vi "Get Package Available Versions.vi"(8 "error in":errorcluster, 11 "package name":string) -> (0 "error out":errorcluster, 2 "versions":string[](array[string]), 3 "package name out":string)   [LabVIEW 2014, in "NIPM_API.lvlib"]
doc: "Returns a list of all the versions (from highest to lowest) of the specified package (in all currently registered feeds on this computer)\n\nINPUT(s)\n<B>Package name</B>: Specifies the package\n\nOUTPUT(s)\n<B>Package name out</B>: Outputs the package name\n\n<B>Versions</B>: Outputs a 1D array that lists all of the available versions of the package from highest to lowest"
uses:
  NIPM_API.lvlib
panel:
  out "cmd standard output":string
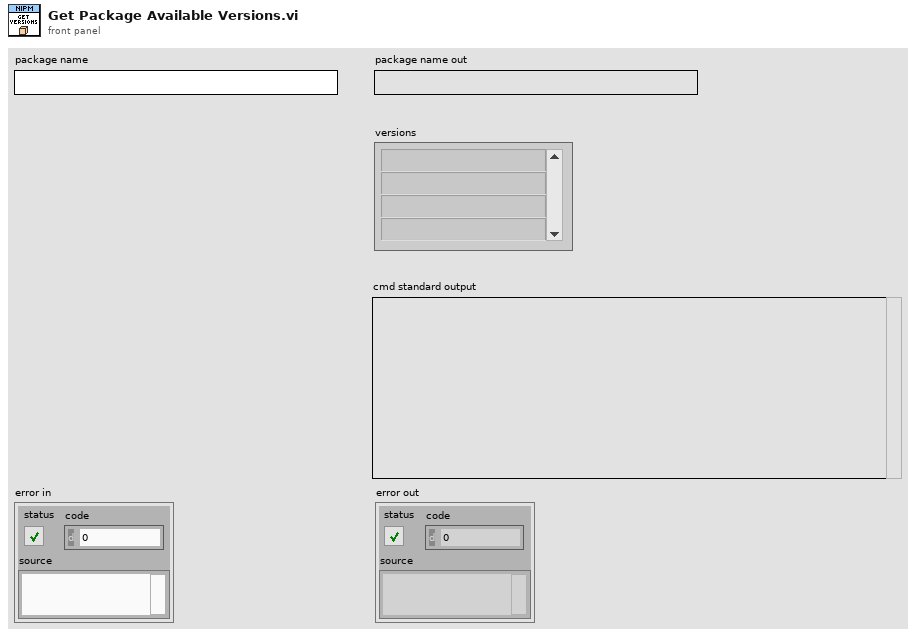
[diagram p1: front panel]
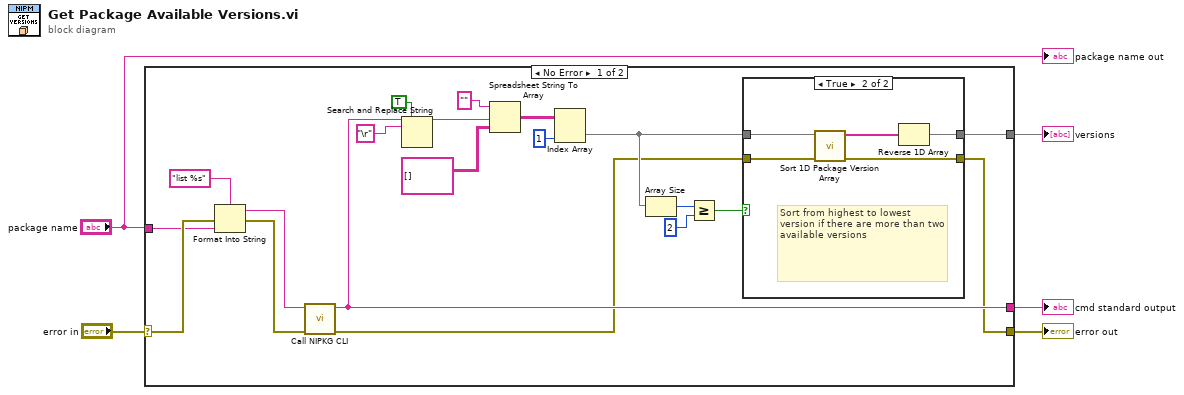
[diagram p0: block diagram]
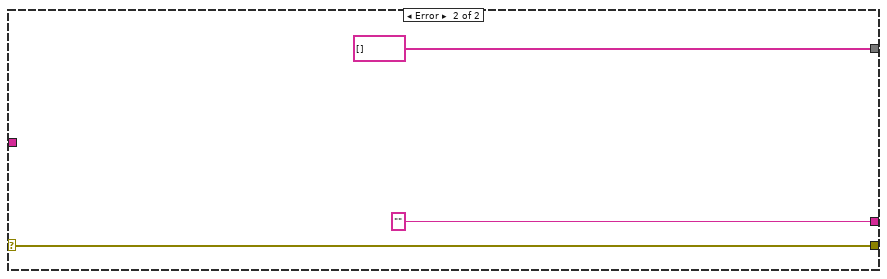
[diagram p3: hidden frame]
diagram:
  n1 = case shown="No Error" "error in" {
    selector: "error in" -> [w24 w35]
    tunnel: [w13 "" ("standard output")] -> w4
    tunnel: [w6 w35] -> w3
    tunnel: [w8 string[] []] -> w2
    tunnel: "package name" -> [w16 _]
    frame No Error {
      n2 = Format Into String(format string="list %s", error in=w24, w16) -> (resulting string=w15:string, error out=w14:errorcluster)  [unwired: 1 in]
      n3 = call "Call NIPKG CLI.vi"("error in (no error)"=w14, "command"=w15) -> ("error out"=w7:errorcluster, "command line standard output"=w13:string)  [unwired: 8 in]
      n4 = Search and Replace String(replace all?=TRUE ("replace all? (F)"), input string=w13, search string="\r") -> (result string=w21:string)  [unwired: 5 in, 3 out]
      n5 = Spreadsheet String To Array(format string="", spreadsheet string=w21, array type (2D Dbl)=string[][] []) -> (array=w18:string[][])  [unwired: 1 in]
      n6 = Index Array(array=w18, index (col)=1 ("disabled index (col)")) -> (element=w9:string[])  [unwired: 1 in]
      n7 = Array Size(array=w9) -> (size(s)=w12:i32)
      n8 = Greater Or Equal?(x=w12, y=2) -> (x >= y?=w10:bool)
      n9 = case shown="True" w10 {
        tunnel: w9 -> [w27 w31]
        tunnel: [w27 w30] -> w8
        tunnel: w7 -> [w26 w29]
        tunnel: [w26 w28] -> w6
        frame False {
        }
        frame True {
          # "Sort from highest to lowest version if there are more than two available versions"
          n10 = call "Sort 1D Package Version Array.vi"("error in (no error)"=w29, "array"=w31) -> ("error out"=w28:errorcluster, "sorted array"=w32:string[])  [unwired: 8 in]
          n11 = Reverse 1D Array(array=w32) -> (reversed array=w30:string[])
        }
      }
    }
    frame Error {
    }
  }
  "error out" <- w3
  "cmd standard output" <- w4
  "versions" <- w2
  "package name out" <- "package name"
